vi "Verifyrollrefcode.vi"() -> ()   [LabVIEW 2019]
uses:
  <vilib>/Platform/TimedLoop/XDataNode/timing_clust.ctl
  <vilib>/Platform/TimedLoop/XDataNode/nitl_modes.ctl
  <vilib>/Platform/TimedLoop/XDataNode/wakeup.ctl
  <vilib>/Utility/file.llb/Read Delimited Spreadsheet (DBL).vi
  <vilib>/platform/TimedLoop/XDataNode/XDataNode.xnode
  <vilib>/Platform/TimedLoop/XDataNode/XDNodeRunTimeDep.lvlib
panel:
  out "Index":i32
  out "Period":i64
  out "Roll Ref":dbl
  out "all rows":dbl[][](array[numeric])
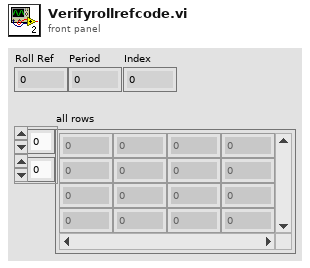
[diagram p1: front panel]
types:
  T1 = typedef "XDNodeRunTimeDep.lvlib/timing_clust.ctl" = cluster{"Expected End [f-1]":u64, "Actual End [f-1]":u64, "Finished Late? [f-1]":bool, "Expected End [i-1]":u64, "Actual End [i-1]":u64, "Finished Late? [i-1]":bool, "Expected Start [i]":u64, "Actual Start [i]":u64, "Expected Start [f]":u64, "Actual Start [f]":u64, "Source Name":string, "Structure Name":string, "Period":i64, "Deadline":i64, "Offset":i64, "Start":i64, "Priority":i32, "Timeout":i32, "Mode":T2, "Wakeup Reason":T3, "Error":errorcluster, "Source Type":string, "Secondary Source Type":string, "Global End Time":u64, "Global Start Time":u64, "Frame Duration":u64, "Iteration Duration":u64, "Assigned CPU":i32, "I/O Scan Engine Mode":u32}
  T2 = typedef "XDNodeRunTimeDep.lvlib/nitl_modes.ctl" = enum32{"No Change", "Process missed periods, maintain original phase", "Discard missed periods, maintain original phase", "Process missed periods, ignore original phase", "Discard missed periods, ignore original phase"}
  T3 = typedef "XDNodeRunTimeDep.lvlib/wakeup.ctl" = enum32{"Normal", "Aborted", "Asynchronous wakeup", "Timing source error", "Timed loop error", "Timeout"}
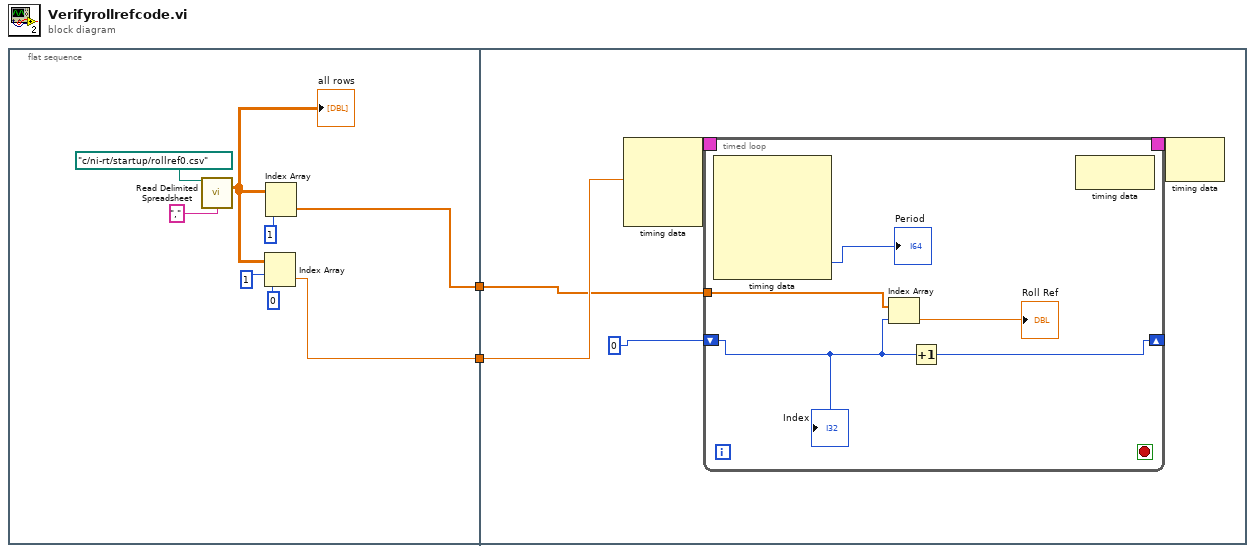
[diagram p0: block diagram]
diagram:
  n1 = flat-sequence {
    tunnel: [w5] -> w2
    tunnel: [w3] -> w1
    tunnel: w2 -> [w12]
    tunnel: w1 -> [w11]
    frame #0 {
      n2 = call-poly <vilib>:"Read Delimited Spreadsheet.vi"("file path (dialog if empty)"=path "c:/ni-rt/startup/rollref0.csv", "delimiter (\\t)"="," ("delimiter (\\t)")) -> ("all rows"=w8:dbl[][])  [unwired: 8 in, 5 out]
      "all rows" <- w8
      n3 = Index Array(array=w8, index (row)=1 ("disabled index (row)"), index (col)=0 ("disabled index (col)")) -> (element=w5:dbl)
      n4 = Index Array(array=w8, index (col)=1) -> (element=w3:dbl[])  [unwired: 1 in]
    }
    frame #1 {
      n5 = node-c288(w12) -> (w15:T1)  [unwired: 3 in]
      n6 = timed-loop {
        timing: w15 -> [_]
        timing-out: [_] -> w14
        shift-right: [w19] -> _
        shift-left: 0 -> [w18]
        tunnel: w11 -> [w16]
        stop <- _ stop-if-true
        n7 = node-c288() -> (→"Period":i64)  [unwired: 1 in, 6 out]
        n8 = Index Array(array=w16, index=w18) -> (element=→"Roll Ref":dbl)
        n9 = Increment(x=w18) -> (x+1=w19:i32)
        n10 = node-c288() -> ()  [unwired: 1 in, 1 out]
        "Index" <- w18
      }
      n11 = node-c288(w14) -> ()  [unwired: 1 out]
    }
  }
